vi "Set Output Values.vi"(8 "Error In":errorcluster, 9 "Start Index":i32, 10 "Values":dbl[](array[numeric]), 11 "BNT_DAQmx-MCSV in":refnum<class "BNT_DAQmx-MCSV.lvclass">=refnum) -> (0 "Error Out":errorcluster, 3 "BNT_DAQmx-MCSV out":refnum<class "BNT_DAQmx-MCSV.lvclass">)   [LabVIEW 2017, in "BNT_DAQmx.lvlib" / "BNT_DAQmx-MCSV.lvclass"]
doc: "Write voltage values to DAQmx device and publish.\n\nTimeout is set to constant 1s."
uses:
  BNT_DAQmx-MCSV.lvclass
  <vilib>/DAQmx/write.llb/DAQmx Write (Analog 1D DBL NChan 1Samp).vi
  CSPP_Core/Classes/CSPP_ProcessVariables/PVConnection/PVConnection.lvclass
  CSPP_Core/Classes/CSPP_ProcessVariables/ProcessVariable/PV.lvclass
  C:/User/Brand/LVP/TASCA/UTCS/Packages/CSPP_Core/Classes/CSPP_BaseClasses/Base/CSPP_Base.lvclass
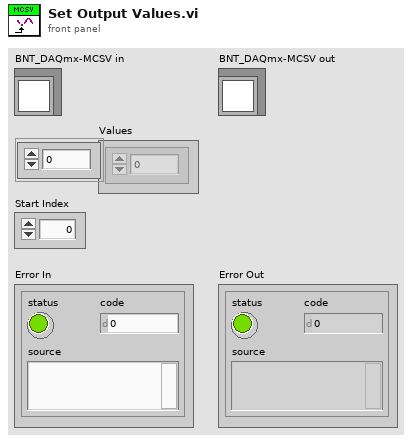
[diagram p1: front panel]
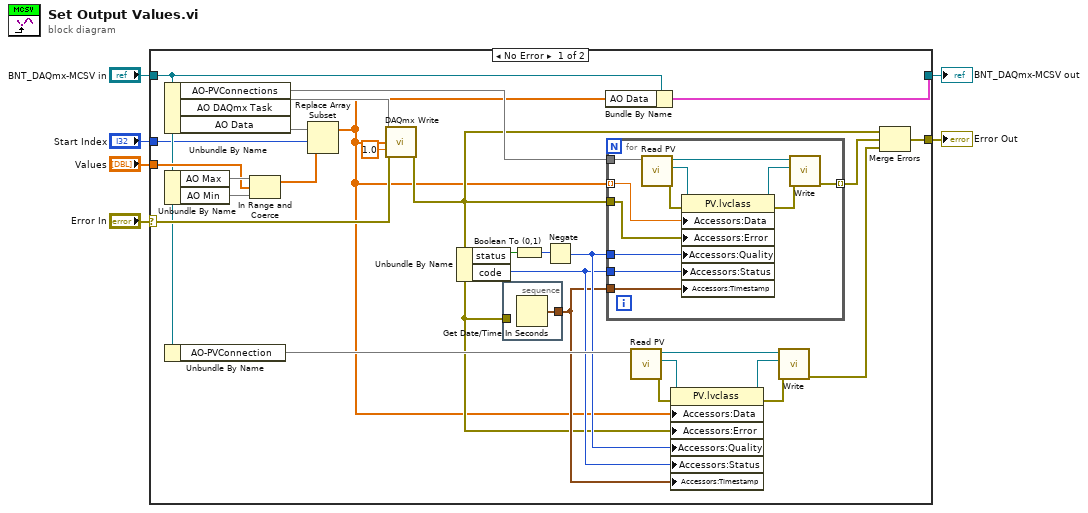
[diagram p0: block diagram]
diagram:
  n1 = case shown="No Error" "Error In" {
    selector: "Error In" -> [w32 w49]
    tunnel: [w28 w49] -> w5
    tunnel: [w23 w48] -> w3
    tunnel: "BNT_DAQmx-MCSV in" -> [w22 w48]
    tunnel: "Values" -> [w24 _]
    tunnel: "Start Index" -> [w7 _]
    frame No Error {
      n2 = Unbundle By Name(w22) -> ("AO-PVConnections"=w27, "AO DAQmx Task"=w34, "AO Data"=w10)
      n3 = Unbundle By Name(w22) -> ("AO Max"=w26, "AO Min"=w25)
      n4 = Unbundle By Name(w22) -> ("AO-PVConnection"=w15)
      n5 = In Range and Coerce(upper limit=w26, x=w24, lower limit=w25) -> (coerced(x)=w9:dbl[])  [unwired: 1 out]
      n6 = Replace Array Subset(array=w10, new element=w9, index=w7) -> (w8:dbl[])
      n7 = call-poly <vilib>:"DAQmx Write.vi"("task/channels in"=w34, "data"=w8, "timeout"=1.0, "error in"=w32) -> ("error out"=w11:errorcluster)  [unwired: 9 in, 2 out]
      n8 = Unbundle By Name(w11) -> ("status"=w30:bool, "code"=w13:i32)
      n9 = stacked-sequence {
        tunnel: [w35] -> w12
        tunnel: w11 -> [_]
        frame #0 {
          n10 = Get Date/Time In Seconds() -> (seconds since 1Jan1904=w35:timestamp)
        }
      }
      n11 = Boolean To (0,1)(Boolean=w30) -> (0, 1=w31:i16)
      n12 = Negate(x=w31) -> (-x=w14:i16)
      n13 = Bundle By Name(cluster=w22, "AO Data"=w8) -> (w23:cluster{})
      n14 = for {
        tunnel: w27 -> [w39]
        tunnel: w8 -> [w47] mode=indexing
        tunnel: w11 -> [w46]
        tunnel: [w43] -> w29 mode=indexing
        tunnel: w14 -> [w42]
        tunnel: w13 -> [w41]
        tunnel: w12 -> [w40]
        n15 = call "Read PV.vi"("PVConnection in"=w39) -> ("error out"=w36:errorcluster, "PV"=w37:refnum<class "PV.lvclass">, "PVConnection out"=w38:refnum<class "PVConnection.lvclass">)  [unwired: 8 in]
        n16 = property class="PV.lvclass"(reference=w37, error in=w36, "Accessors:Data"=w47, "Accessors:Error"=w46, "Accessors:Quality"=w42, "Accessors:Status"=w41, "Accessors:Timestamp"=w40) -> (reference out=w45:refnum<class "PV.lvclass">, error out=w44:errorcluster)
        n17 = call "Write.vi"("error in (no error)"=w44, "PV"=w45, "PVConnection in"=w38) -> ("error out"=w43:errorcluster)  [unwired: 7 in, 1 out]
      }
      n18 = call "Read PV.vi"("PVConnection in"=w15) -> ("error out"=w21:errorcluster, "PV"=w20:refnum<class "PV.lvclass">, "PVConnection out"=w19:refnum<class "PVConnection.lvclass">)  [unwired: 8 in]
      n19 = property class="PV.lvclass"(reference=w20, error in=w21, "Accessors:Data"=w8, "Accessors:Error"=w11, "Accessors:Quality"=w14, "Accessors:Status"=w13, "Accessors:Timestamp"=w12) -> (reference out=w17:refnum<class "PV.lvclass">, error out=w18:errorcluster)
      n20 = call "Write.vi"("error in (no error)"=w18, "PV"=w17, "PVConnection in"=w19) -> ("error out"=w16:errorcluster)  [unwired: 7 in, 1 out]
      n21 = Merge Errors(w11, w29, w16) -> (w28:errorcluster)
    }
    frame Error {
    }
  }
  "Error Out" <- w5
  "BNT_DAQmx-MCSV out" <- w3
